vi "notifyObservers.vi"(8 "error in (no error)":errorcluster, 11 "WeatherData in":refnum<class "WeatherData.lvclass">) -> (0 "error out":errorcluster, 3 "WeatherData out":refnum<class "WeatherData.lvclass">)   [LabVIEW 2017, in "WeatherData.lvclass"]
uses:
  WeatherData.lvclass
  Observer/Observer.lvclass
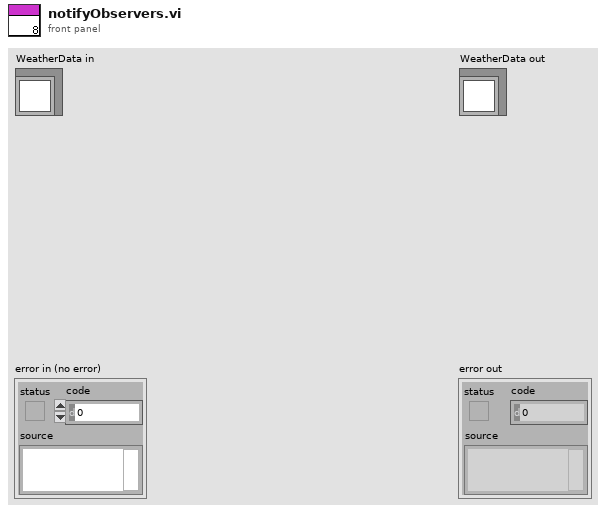
[diagram p1: front panel]
types:
  T1 = cluster{"Temperature":dbl, "Humidity":dbl, "Pressure":dbl, "Stop?":bool}
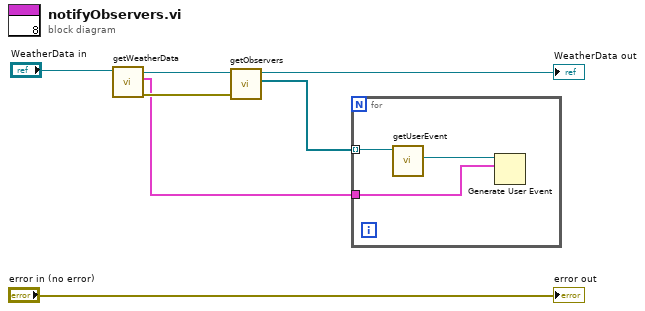
[diagram p0: block diagram]
diagram:
  n1 = call-dynamic "getWeatherData.vi"("WeatherData in"="WeatherData in") -> ("error out"=w5:errorcluster, "WeatherData"=w3:T1, "WeatherData out"=w6:refnum<class "WeatherData.lvclass">)  [unwired: 8 in]
  n2 = call-dynamic "getObservers.vi"("error in (no error)"=w5, "WeatherData in"=w6) -> ("Observers"=w4:refnum<class "Observer.lvclass">[], "WeatherData out"=→"WeatherData out":refnum<class "WeatherData.lvclass">)  [unwired: 7 in, 1 out]
  n3 = for {
    tunnel: w4 -> [w10] mode=indexing
    tunnel: w3 -> [w8]
    n4 = call-dynamic "getUserEvent.vi"("Observer in"=w10) -> ("UserEvent"=w9:refnum<user-event>)  [unwired: 8 in, 2 out]
    n5 = Generate User Event(user event=w9, event data cluster=w8) -> ()  [unwired: 2 in, 2 out]
  }
  "error out" <- "error in (no error)"
